vi "isNanOrInf.vi"(0 "Utilities in":refnum<class "Utilities.lvclass">, 1 "value":dbl format="%#_13g", 5 "error in (no error)":errorcluster) -> (14 "Utilities out":refnum<class "Utilities.lvclass">, 15 "nan?":bool, 16 "+inf?":bool, 17 "-inf?":bool, 18 "narOrInf?":bool, 19 "error out":errorcluster)   [LabVIEW 2023, in "Utilities.lvclass"]
uses:
  Utilities.lvclass
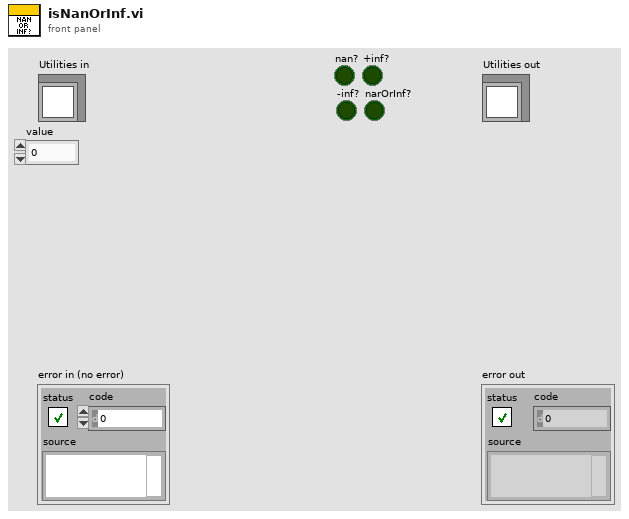
[diagram p1: front panel]
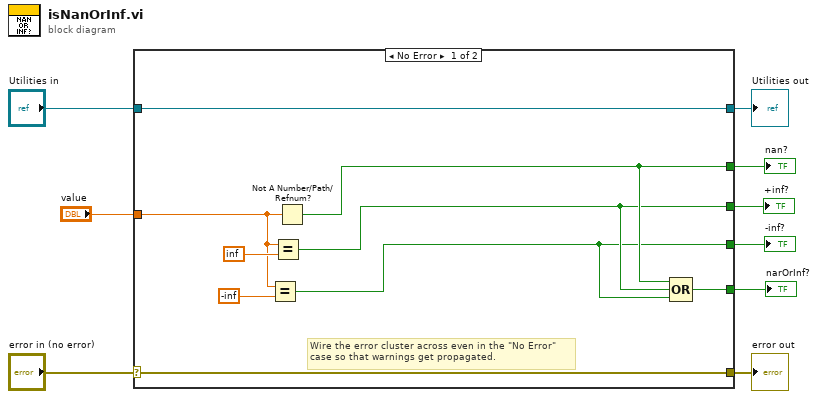
[diagram p0: block diagram]
diagram:
  n1 = case shown="No Error" "error in (no error)" {
    selector: "error in (no error)" -> [w17 w20]
    tunnel: [w17 w20] -> w8
    tunnel: [w18 w19] -> w6
    tunnel: "Utilities in" -> [w18 w19]
    tunnel: "value" -> [w14 _]
    tunnel: [w13 _] -> w4
    tunnel: [w12 _] -> w3
    tunnel: [w11 _] -> w2
    tunnel: [w10 _] -> w1
    frame No Error {
      # "Wire the error cluster across even in the \"No Error\"\ncase so that warnings get propagated."
      n2 = Equal?(x=w14, y=-inf) -> (x = y?=w11:bool)
      n3 = Equal?(x=w14, y=inf) -> (x = y?=w12:bool)
      n4 = Not A Number/Path/Refnum?(number/path/refnum=w14) -> (NaN/Path/Refnum?=w13:bool)
      n5 = Compound Arithmetic op=OR(w13, w12, w11) -> (w10:bool)
    }
    frame Error {
    }
  }
  "error out" <- w8
  "Utilities out" <- w6
  "nan?" <- w4
  "+inf?" <- w3
  "-inf?" <- w2
  "narOrInf?" <- w1
